vi "Option Recognition.vi"(8 "error in (no error)":errorcluster, 10 "Option (\"\")":string, 11 "VISA resource name":refnum<visa-resource-name>) -> (0 "error out":errorcluster, 2 "Is Option Installed":bool, 3 "VISA resource name out":refnum<visa-resource-name>)   [LabVIEW 2018, in "Agilent PSG MXG Series.lvlib"]
doc: "Specifies whether the option is installed."
uses:
  Agilent PSG MXG Series.lvlib
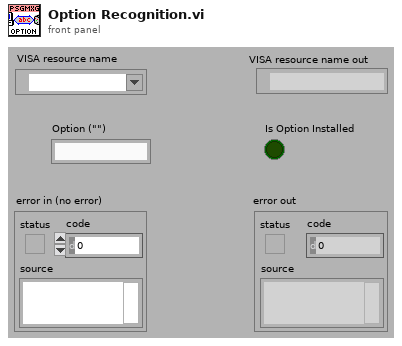
[diagram p1: front panel]
types:
  T1 = typedef "Agilent PSG MXG Series.lvlib/Extended User Data.ctl" = cluster{"Options":string[]}
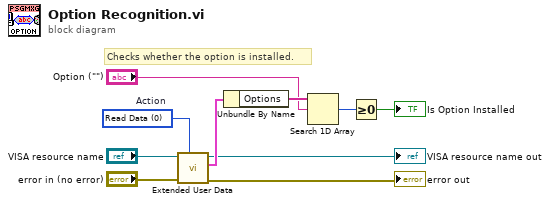
[diagram p0: block diagram]
diagram:
  w8 = u16 0 items=["Read Data", "Write Data", "Clear Data", "Clear ALL Data"]  # Action
  # "Checks whether the option is installed."
  n1 = call "Extended User Data.vi"("Action"=w8, "error in (no error)"="error in (no error)", "VISA resource name"="VISA resource name") -> ("error out"=→"error out":errorcluster, "User Data Out"=w7:T1, "VISA resource name out"=→"VISA resource name out":refnum<visa-resource-name>)  [unwired: 1 in, 5 out]
  n2 = Unbundle By Name(w7) -> ("Options"=w6:string[])
  n3 = Search 1D Array(1D array=w6, element="Option (\"\")") -> (index of element=w4:i32)  [unwired: 1 out]
  n4 = Greater Or Equal To 0?(x=w4) -> (x >= 0?=→"Is Option Installed":bool)
